vi "Encode P2P CAN-ID.vi"(10 "COB Peer-To-Peer":T1 items=["EMCY"=1, "PDO1 (tx)"=3, "PDO1 (rx)"=4, "PDO2 (tx)"=5, "PDO2 (rx)"=6, "PDO3 (tx)"=7, "PDO3 (rx)"=8, "PDO4 (tx)"=9, "PDO4 (rx)"=10, "SDO (tx)"=11, "SDO (rx)"=12, "NMT error control"=14], 11 "Node ID":u8) -> (3 "CAN-ID":u32 format="%.0x")   [LabVIEW 2024, in "CANopen.lvlib" / "CANopen.lvclass"]
doc: "Combines the function code and the node ID into CAN-ID"
uses:
  CANopen.lvclass
  COB Peer-To-Peer.ctl
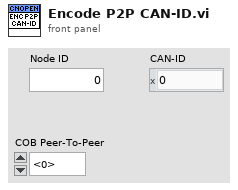
[diagram p1: front panel]
types:
  T1 = typedef "COB Peer-To-Peer.ctl" = u16
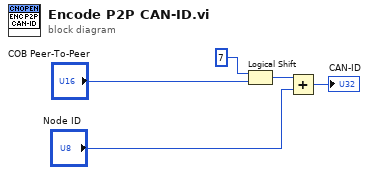
[diagram p0: block diagram]
diagram:
  n1 = Logical Shift(y=i16 7, x="COB Peer-To-Peer") -> (x << y=w4:T1)
  n2 = Add(x=w4, y="Node ID") -> (x+y=→"CAN-ID":T1)
